vi "OAT Slow Roll Compensation.vi"(4 "number of rev to average":i32, 6 "slow roll rev index":i32, 7 "reset? (True)":bool=TRUE, 8 "error in (no error)":errorcluster, 10 "baseline in":cluster{"r0":dbl, "dr":dbl, "Y":dbl[]}={"r0"=0.0, "dr"=1.0, "Y"=[]} {"r0" format="%.2p"; "dr" format="%.2p"; "Y" format="%.2f"}, 11 "resampled signal":cluster{"r0":dbl, "dr":dbl, "Y":dbl[]}={"r0"=0.0, "dr"=1.0, "Y"=[]} {"r0" format="%.2p"; "dr" format="%.2p"; "Y" format="%.2f"}) -> (0 "error out":errorcluster, 2 "baseline out":cluster{"r0":dbl, "dr":dbl, "Y":dbl[]}={"r0"=0.0, "dr"=1.0, "Y"=[]} {"r0" format="%.2p"; "dr" format="%.2p"; "Y" format="%.2f"}, 3 "compensated signal":cluster{"r0":dbl, "dr":dbl, "Y":dbl[]}={"r0"=0.0, "dr"=1.0, "Y"=[]} {"r0" format="%.2p"; "dr" format="%.2p"; "Y" format="%.2f"})   [LabVIEW 2017]
doc: "Remove the slow roll baseline from the <B>resampled signal</B>, so that only the dynamic response remains. This VI can be used for continuous processing. When running for the first data block, <B>reset? (True)</B> should be set to True. The slowroll baseline can be provided by either <B>baseline in</B> or specifying the slow roll range in terms of <B>slow rool rev index</B> and <B>number of rev to average</B>. In the latter situation, the VI will automatically generates the slow roll baseline."
uses:
  <vilib>/addons/Sound and Vibration/Order Analysis/Resample Order Tracking/SubVIs/OAT Verify Resampled Signal (Single Channel).vi
  <vilib>/addons/Sound and Vibration/Order Analysis/Resample Order Tracking/SoundVib_Resampling.lvlib
panel:
  # "OAT Slow Roll Compensation"
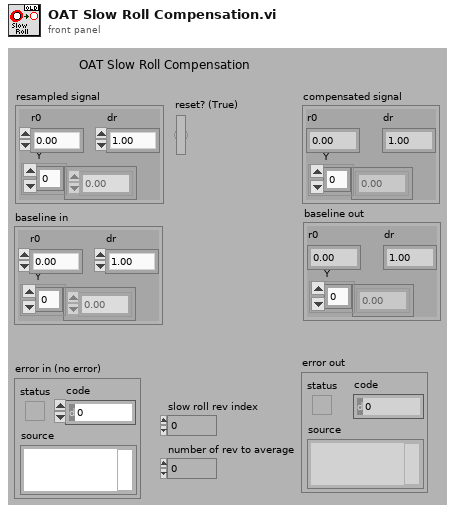
[diagram p1: front panel]
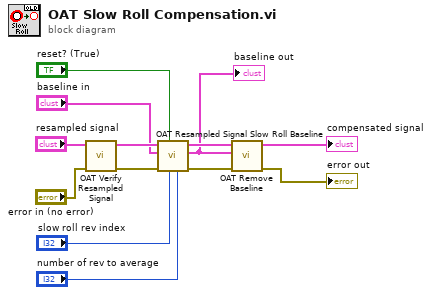
[diagram p0: block diagram]
diagram:
  n1 = call-poly <vilib>:"OAT Verify Resampled Signal.vi"("error in (no error)"="error in (no error)", "resampled signal"="resampled signal") -> ("error out"=w7:errorcluster, "resampled signal dup"=w9:cluster{"r0":dbl, "dr":dbl, "Y":dbl[]})  [unwired: 7 in, 1 out]
  n2 = call <vilib>:"OAT Resampled Signal Slow Roll Baseline.vi"("average revolution"="number of rev to average", "slow roll\nrevolution number"="slow roll rev index", "reset? (True)"="reset? (True)", "error in (no error)"=w7, "baseline in"="baseline in", "resampled signal in"=w9) -> ("error out"=w6:errorcluster, "baseline out"=w1:cluster{"r0":dbl, "dr":dbl, "Y":dbl[]}, "resampled signal out"=w8:cluster{"r0":dbl, "dr":dbl, "Y":dbl[]})  [unwired: 3 in]
  "baseline out" <- w1
  n3 = call <vilib>:"OAT Remove Baseline.vi"("error in (no error)"=w6, "baseline in"=w1, "resampled signal in"=w8) -> ("error out"=→"error out":errorcluster, "compensated signal"=→"compensated signal":cluster{"r0":dbl, "dr":dbl, "Y":dbl[]})  [unwired: 7 in]
